vi "Print.vi"(11 "Ref In":refnum<k7>) -> ()   [LabVIEW 2018]
panel:
  # "PRINT"
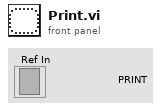
[diagram p1: front panel]
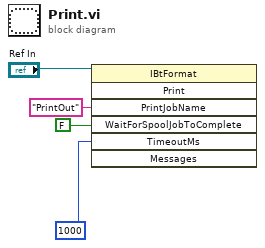
[diagram p0: block diagram]
diagram:
  n1 = invoke class="IBtFormat" method="Print"(reference="Ref In", "PrintJobName"="PrintOut", "WaitForSpoolJobToComplete"=FALSE, "TimeoutMs"=1000) -> ()  [unwired: 3 in, 7 out]
